vi "unmarshalling.vi"(7 "Type":variant, 8 "error in (no error)":errorcluster, 10 "String":string, 11 "Serializer in":refnum<class "Serializer.Template.lvclass">) -> (0 "error out":errorcluster, 2 "Variant":variant, 3 "Serializer":refnum<class "Serializer.Template.lvclass">)   [LabVIEW 2013, in "OpenSerializer.Template.lvlib" / "Serializer.Template.lvclass"]
uses:
  Serializer.Template.lvclass
  <vilib>/LabVIEW Open Source Project/OpenSerializer/Serializer/Serializer.lvclass
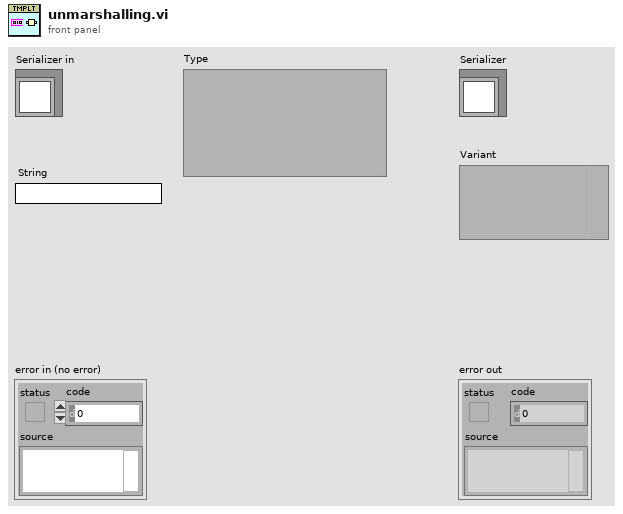
[diagram p1: front panel]
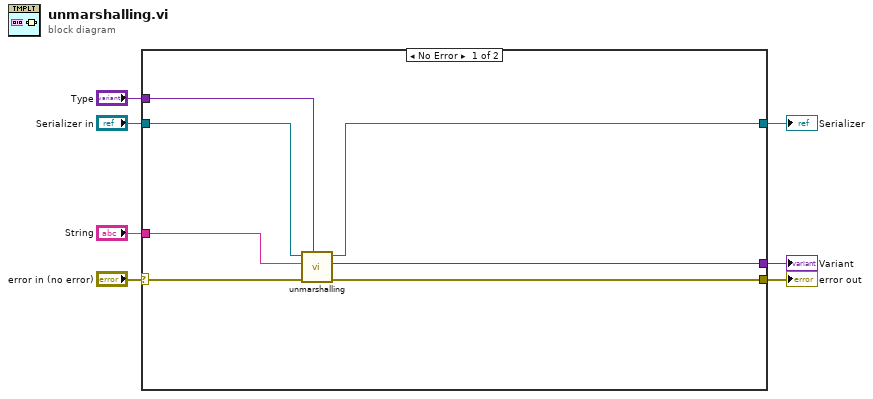
[diagram p0: block diagram]
diagram:
  n1 = case shown="No Error" "error in (no error)" {
    selector: "error in (no error)" -> [w10 w15]
    tunnel: "Serializer in" -> [w14 w16]
    tunnel: "String" -> [w11 _]
    tunnel: [w12 w16] -> w5
    tunnel: [w9 w15] -> w4
    tunnel: [w8 _] -> w3
    tunnel: "Type" -> [w13 _]
    frame No Error {
      n2 = call-parent "unmarshalling.vi"("Type"=w13, "error in (no error)"=w10, "String"=w11, "Serializer in"=w14) -> ("error out"=w9:errorcluster, "Variant"=w8:variant, "Serializer out"=w12:refnum<class "Serializer.Template.lvclass">)  [unwired: 5 in]
    }
    frame Error {
    }
  }
  "error out" <- w4
  "Serializer" <- w5
  "Variant" <- w3
